vi "Get System Name.vi"() -> (3 "name":string)   [LabVIEW 2023, in "Logger.lvclass"]
uses:
  logger/Logger.lvclass
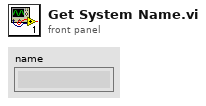
[diagram p1: front panel]
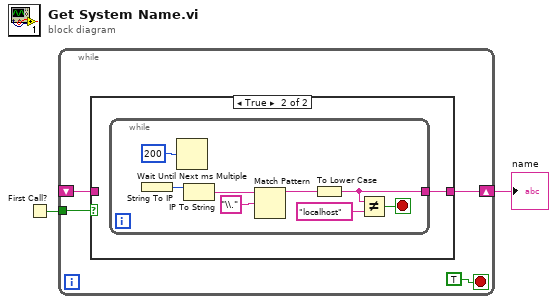
[diagram p0: block diagram]
diagram:
  n1 = First Call?() -> (First Call?: T/F=w1:bool)
  n2 = while {
    tunnel: w1 -> [w5]
    shift-right: [w6] -> w2
    shift-left: _ -> [w3]
    stop <- TRUE stop-if-true
    n3 = case shown="True" w5 {
      tunnel: [w7 w8] -> w6
      tunnel: w3 -> [w7 _]
      frame False {
      }
      frame True {
        n4 = while {
          tunnel: [w9] -> w8
          stop <- w14 stop-if-true
          n5 = String To IP() -> (0:w16:u32)  [unwired: 1 in]
          n6 = Wait Until Next ms Multiple(millisecond multiple=u32 200) -> ()  [unwired: 1 out]
          n7 = IP To String(2:w16) -> (0:w11:string)  [unwired: 1 in]
          n8 = Match Pattern(string=w11, regular expression="\\.") -> (before substring=w10:string)  [unwired: 1 in, 3 out]
          n9 = To Lower Case(string=w10) -> (all lower case string=w9:string)
          n10 = Not Equal?(x=w9, y="localhost") -> (x != y?=w14:bool)
        }
      }
    }
  }
  "name" <- w2
